vi "finish.vi"(8 "ErrorIn":errorcluster, 11 "QueuesIn":T1) -> (0 "ErrorOut":errorcluster)   [LabVIEW 2019]
uses:
  utilities/AQueues.ctl
  AmasterVIs/ACommand.ctl
  analyzeAccelerationDataVIs/AccelerationDataFrames.ctl
  analyzeAccelerationDataVIs/AnalyzedVibrationsData.ctl
  analyzeAccelerationDataVIs/calculateFaultIndicatorsVIs/FaultDetections.ctl
  analyzeAccelerationDataVIs/calculateFaultIndicatorsVIs/ParameterFaultDetection.ctl
  analyzeAccelerationDataVIs/calculateFaultIndicatorsVIs/FaultParameter.ctl
  analyzeAccelerationDataVIs/calculateFaultIndicatorsVIs/FrequencyFaultDetection.ctl
  TDMSmanagerVIs/TDMSAnalyzerData.ctl
  TDMSmanagerVIs/TDMSAnalyzerDataType.ctl
  AmasterVIs/ACommandQueuesAction.ctl
  <vilib>/myRIO/Common/Instrument Driver Framework/myRIO v1.0/UART/vis/myRIO v1.0 Close UART.vi
  <vilib>/myRIO/Common/Instrument Driver Framework/Utilities/vis/FPGA Ref Manager.vi
  <vilib>/myRIO/Common/Instrument Driver Framework/myRIO v1.0/myRIO v1.0 Reset FPGA.vi
  <vilib>/myRIO/Common/Instrument Driver Framework/myRIO v1.0/IRQ/vis/myRIO v1.0 IRQ Info FGV.vi
  <vilib>/myRIO/Common/Instrument Driver Framework/myRIO v1.0/IRQ/vis/myRIO v1.0 Timer IRQ Info FGV.vi
  <vilib>/myRIO/Common/Instrument Driver Framework/myRIO v1.0/IRQ/vis/myRIO v1.0 ISR Agent.vi
  <vilib>/myRIO/Instrument Drivers/Utilities/vis/Reset Index.vi
  <vilib>/myRIO/Common/Instrument Driver Framework/myRIO v1.0/Resource Manager/vis/myRIO v1.0 Block Write Resource Manager.vi
  <vilib>/myRIO/Instrument Drivers/Utilities/Utilities.lvlib
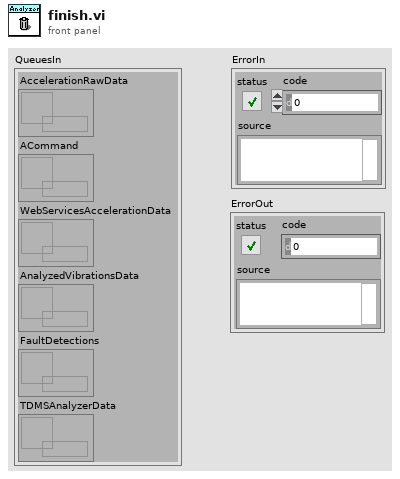
[diagram p1: front panel]
types:
  T1 = typedef "AQueues.ctl" = cluster{"AccelerationRawData":refnum<queue>, "ACommand":refnum<queue>, "WebServicesAccelerationData":refnum<queue>, "AnalyzedVibrationsData":refnum<queue>, "FaultDetections":refnum<queue>, "TDMSAnalyzerData":refnum<queue>}
  T2 = typedef "ACommandQueuesAction.ctl" = enum16{"Initialize", "Set", "Get", "ReleaseAll"}
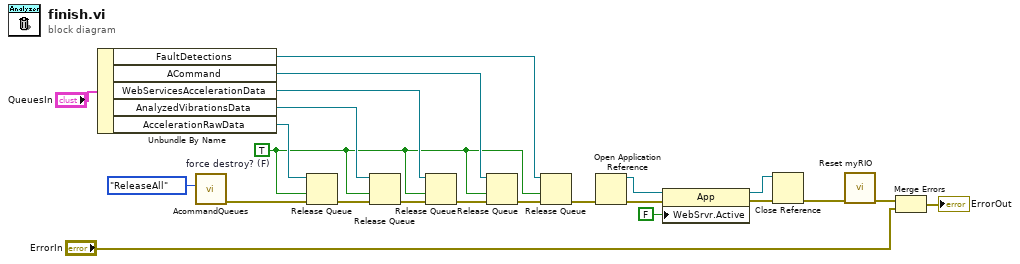
[diagram p0: block diagram]
diagram:
  w2 = TRUE  # force destroy? (F)
  n1 = Unbundle By Name("QueuesIn") -> ("FaultDetections"=w3:refnum<queue>, "ACommand"=w5:refnum<queue>, "WebServicesAccelerationData"=w18:refnum<queue>, "AnalyzedVibrationsData"=w20:refnum<queue>, "AccelerationRawData"=w22:refnum<queue>)
  n2 = call "AcommandQueues.vi"("ACommandQueuesAction"=ACommandQueuesAction."ReleaseAll") -> ("ErrorOut"=w11:errorcluster)  [unwired: 9 in, 1 out]
  n3 = Release Queue(queue=w22, force destroy? (F)=w2, error in (no error)=w11) -> (error out=w21:errorcluster)  [unwired: 2 out]
  n4 = Release Queue(queue=w20, force destroy? (F)=w2, error in (no error)=w21) -> (error out=w19:errorcluster)  [unwired: 2 out]
  n5 = Release Queue(queue=w18, force destroy? (F)=w2, error in (no error)=w19) -> (error out=w6:errorcluster)  [unwired: 2 out]
  n6 = Release Queue(queue=w5, force destroy? (F)=w2, error in (no error)=w6) -> (error out=w4:errorcluster)  [unwired: 2 out]
  n7 = Release Queue(queue=w3, force destroy? (F)=w2, error in (no error)=w4) -> (error out=w1:errorcluster)  [unwired: 2 out]
  n8 = Open Application Reference(8:w1) -> (0:w17:errorcluster, 3:w16:refnum<vi>)  [unwired: 3 in]
  n9 = property class="App"(reference=w16, error in=w17, "WebSrvr.Active"=FALSE ("Web Server:Server Active")) -> (reference out=w13:refnum<vi>, error out=w14:errorcluster)
  n10 = Close Reference(reference=w13, error in (no error)=w14) -> (error out=w12:errorcluster)
  n11 = call <vilib>:"Reset myRIO.vi"("error in (no error)"=w12) -> ("error out"=w9:errorcluster)  [unwired: 10 in]
  n12 = Merge Errors(w9, "ErrorIn") -> (→"ErrorOut":errorcluster)
